vi "dfd_Check Filter Set Index.vi"(7 "#filter sets":i32, 8 "error in (no error)":errorcluster, 11 "filter set index in":i32) -> (0 "error out":errorcluster, 3 "filter set index out":i32)   [LabVIEW 2017, in "NI_DigFilter_CodeGen.lvlib"]
uses:
  <vilib>/addons/Digital Filter Design/NI_DigFilter_CodeGen.lvlib
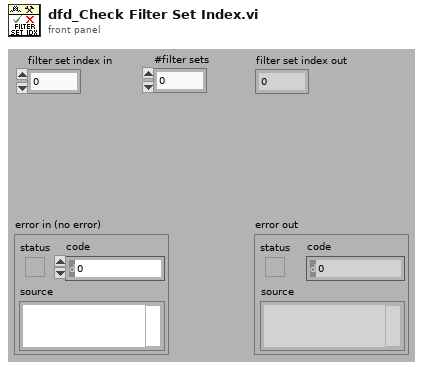
[diagram p1: front panel]
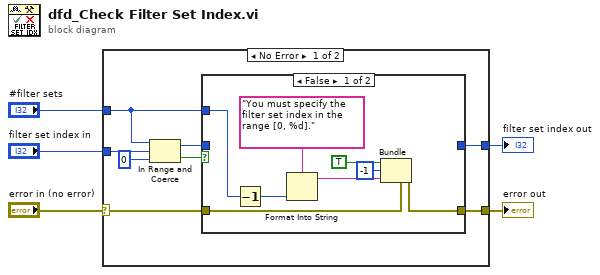
[diagram p0: block diagram]
diagram:
  n1 = case shown="No Error" "error in (no error)" {
    selector: "error in (no error)" -> [w11 w24]
    tunnel: "#filter sets" -> [w6 _]
    tunnel: "filter set index in" -> [w12 _]
    tunnel: [w8 _] -> w2
    tunnel: [w7 w24] -> w1
    frame No Error {
      n2 = In Range and Coerce(upper limit=w6, x=w12, lower limit=0) -> (coerced(x)=w9:i32, In Range?=w10:bool)
      n3 = case shown="False" w10 {
        tunnel: w11 -> [w21 w22]
        tunnel: w9 -> [_ w23]
        tunnel: [_ w23] -> w8
        tunnel: [w20 w22] -> w7
        tunnel: w6 -> [w16 _]
        frame False {
          n4 = Decrement(x=w16) -> (x-1=w14:i32)
          n5 = Format Into String(format string="You must specify the filter set index in the range [0, %d].", w14) -> (resulting string=w15:string)  [unwired: 2 in, 1 out]
          n6 = Bundle(cluster=w21, "status"=TRUE, "code"=-1, "source"=w15) -> (w20:errorcluster)
        }
        frame True {
        }
      }
    }
    frame Error {
    }
  }
  "error out" <- w1
  "filter set index out" <- w2
